vi "Add Unknown Type.vi"(0 "JSON Tree out (JSON Object) in":variant, 5 "result":variant, 9 "Name":string, 11 "error in (no error)":errorcluster) -> (4 "JSON Tree out (JSON Object) out":variant, 15 "error out":errorcluster)   [LabVIEW 2017, in "JSON_RPC_client.lvlib"]
uses:
  JSON_RPC_client.lvlib
  <vilib>/LVH/i3 JSON/JSON Generation/Add Object Parameter Files/Add Object Parameter - String.vi
  <vilib>/LVH/i3 JSON/JSON Generation/Add Object Parameter Files/Add Object Parameter - Object.vi
  <vilib>/LVH/i3 JSON/JSON Generation/Add Object Parameter Files/Add Object Parameter - Array.vi
  <vilib>/LVH/i3 JSON/JSON Generation/Add Object Parameter Files/Add Object Parameter - Boolean.vi
  <vilib>/LVH/i3 JSON/JSON Generation/Add Object Parameter Files/Add Object Parameter - Numeric.vi
  <vilib>/LVH/i3 JSON/JSON Generation/Add Object Parameter Files/Add Object Parameter - 1D Array Boolean.vi
  <vilib>/LVH/i3 JSON/JSON Generation/Add Object Parameter Files/Add Object Parameter - 1D Array String.vi
  <vilib>/LVH/i3 JSON/JSON Generation/Add Object Parameter Files/Add Object Parameter - 1D Array Double.vi
  <vilib>/Utility/Data Type/NI_Data Type.lvlib
  <vilib>/LVH/i3 JSON/i3-json.lvlib
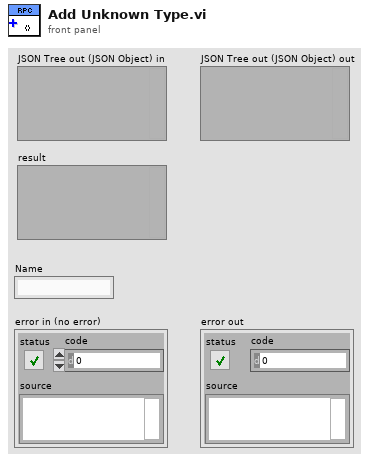
[diagram p1: front panel]
types:
  T1 = typedef "NI_Data Type.lvlib/Data Type.ctl" = enum8{"Invalid Type", "Void", "I8", "I16", "I32", "I64", "U8", "U16", "U32", "U64", "Single Float", "Double Float", "Extended Float", "Single Complex", "Double Complex", "Extended Complex", "Enum U8", "Enum U16", "Enum U32", "Enum U64", "Single Float With Unit", "Double Float With Unit", "Extended Float With Unit", "Single Complex with Unit", "Double Complex with Unit", "Extended Complex with Unit", "Boolean", "String", "Path", "Picture", "Tag", "Array", "Cluster", "Variant", "LV Variant", "Waveform", "Timestamp", "Digital Waveform", "Digital Data", "ExpressData", "Refnum", "External Data", "VI", "Poly VI", "LabVIEW Class Instance", "Fixed Point"}
  T2 = typedef "i3-json.lvlib/JSON Compatible Type.ctl" = enum16{"1D Double Array", "1D String Array", "1D Boolean Array", "Unknown"}
  T3 = typedef "i3-json.lvlib/JSON Type.ctl" = enum8{"JSON Compatible", "JSON Array", "JSON Object", "JSON Null", "Double", "String", "Boolean", "Unknown"}
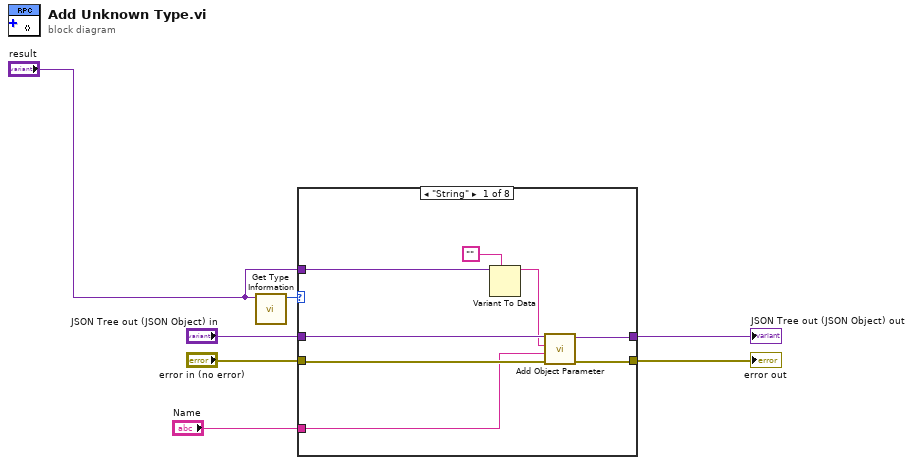
[diagram p0: block diagram]
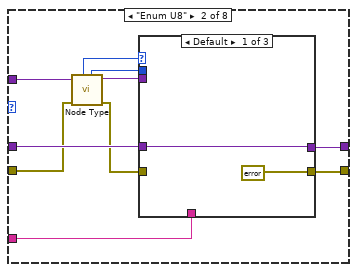
[diagram p2: hidden frame]
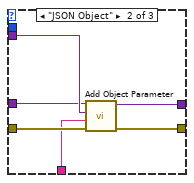
[diagram p3: hidden frame]
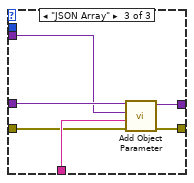
[diagram p4: hidden frame]
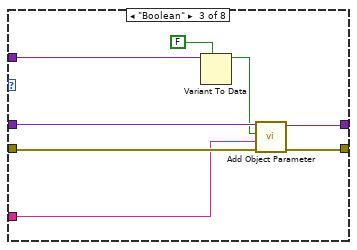
[diagram p5: hidden frame]
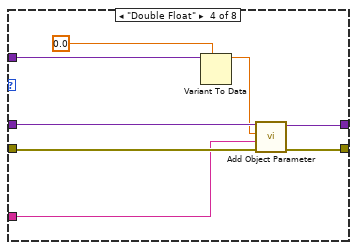
[diagram p6: hidden frame]
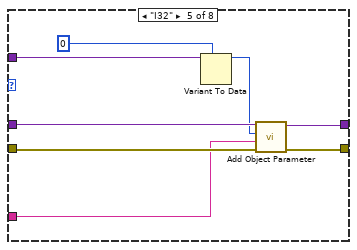
[diagram p7: hidden frame]
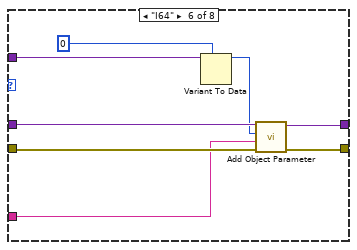
[diagram p8: hidden frame]
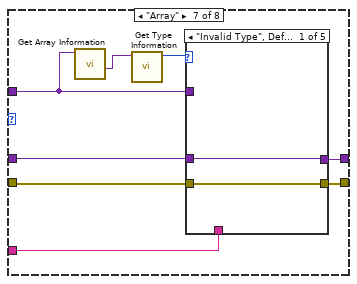
[diagram p9: hidden frame]
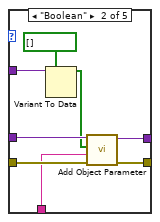
[diagram p10: hidden frame]
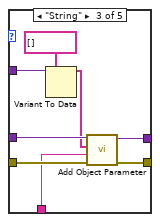
[diagram p11: hidden frame]
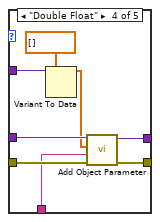
[diagram p12: hidden frame]
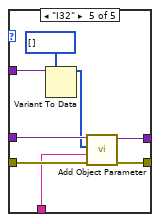
[diagram p13: hidden frame]
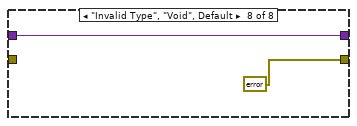
[diagram p14: hidden frame]
diagram:
  n1 = call <vilib>:"Get Type Information.vi"("Variant"="result") -> ("Type"=w6:T1)  [unwired: 6 in, 4 out]
  n2 = case shown="\"String\"" w6 {
    tunnel: "error in (no error)" -> [w12 w20 w44 w52 w60 w68 w76 _]
    tunnel: "JSON Tree out (JSON Object) in" -> [w15 w25 w47 w55 w63 w71 w79 w114]
    tunnel: [w14 w24 w46 w54 w62 w70 w78 w114] -> w3
    tunnel: [w13 w23 w45 w53 w61 w69 w77 errorcluster {"status"=TRUE, "code"=-32603, "source"="JSON-RPC error.  Internal Error.  Result unable to format into JSON.  Ensure the result data type is JSON Object,String, Double, I32, Boolean, or arrays of the same"} ("error constant")] -> w4
    tunnel: "Name" -> [w11 w22 w43 w51 w59 w67 w75 _]
    tunnel: "result" -> [w10 w21 w42 w50 w58 w66 w74 _]
    frame "String" {
      n3 = Variant To Data(type="", Variant=w10) -> (data=w8:string)  [unwired: 1 in, 1 out]
      n4 = call-poly <vilib>:"Add Object Parameter.vi"("error in (no error)"=w12, "Name"=w11, "String"=w8, "JSON Tree in (JSON Object)"=w15) -> ("error out"=w13:errorcluster, "JSON Tree out (JSON Object)"=w14:variant)  [unwired: 6 in]
    }
    frame "Enum U8" {
      n5 = call <vilib>:"Node Type.vi"("error in (no error)"=w20, "JSON Tree In"=w21) -> ("error out"=w19:errorcluster, "JSON Tree Passthrough"=w16:variant, "JSON Compatible Type"=w17:T2, "JSON Type"=w18:T3)  [unwired: 5 in, 1 out]
      n6 = case shown="Default" w18 {
        tunnel: w25 -> [w26 w31 w39]
        tunnel: [w26 w30 w38] -> w24
        tunnel: [errorcluster {"status"=TRUE, "code"=-32603, "source"="JSON-RPC error.  Internal Error.  Result unable to format into JSON.  Ensure the reult data type is JSON Object,String, Double, I32, Boolean, or arrays of the same"} ("error constant") w29 w37] -> w23
        tunnel: w22 -> [_ w28 w36]
        tunnel: w19 -> [_ w33 w35]
        tunnel: w17 -> [_ _ _]
        tunnel: w16 -> [_ w32 w34]
        frame Default {
        }
        frame "JSON Object" {
          n7 = call-poly <vilib>:"Add Object Parameter.vi"("error in (no error)"=w33, "Name"=w28, "JSON Object"=w32, "JSON Tree in (JSON Object)"=w31) -> ("error out"=w29:errorcluster, "JSON Tree out (JSON Object)"=w30:variant)  [unwired: 6 in]
        }
        frame "JSON Array" {
          n8 = call-poly <vilib>:"Add Object Parameter.vi"("error in (no error)"=w35, "Name"=w36, "JSON Array"=w34, "JSON Tree in (JSON Object)"=w39) -> ("error out"=w37:errorcluster, "JSON Tree out (JSON Object)"=w38:variant)  [unwired: 6 in]
        }
      }
    }
    frame "Boolean" {
      n9 = Variant To Data(type=FALSE, Variant=w42) -> (data=w40:bool)  [unwired: 1 in, 1 out]
      n10 = call-poly <vilib>:"Add Object Parameter.vi"("error in (no error)"=w44, "Name"=w43, "Boolean"=w40, "JSON Tree in (JSON Object)"=w47) -> ("error out"=w45:errorcluster, "JSON Tree out (JSON Object)"=w46:variant)  [unwired: 6 in]
    }
    frame "Double Float" {
      n11 = Variant To Data(type=0.0, Variant=w50) -> (data=w48:dbl)  [unwired: 1 in, 1 out]
      n12 = call-poly <vilib>:"Add Object Parameter.vi"("error in (no error)"=w52, "Name"=w51, "Numeric"=w48, "JSON Tree in (JSON Object)"=w55) -> ("error out"=w53:errorcluster, "JSON Tree out (JSON Object)"=w54:variant)  [unwired: 6 in]
    }
    frame "I32" {
      n13 = Variant To Data(type=0, Variant=w58) -> (data=w56:i32)  [unwired: 1 in, 1 out]
      n14 = call-poly <vilib>:"Add Object Parameter.vi"("error in (no error)"=w60, "Name"=w59, "Numeric"=w56, "JSON Tree in (JSON Object)"=w63) -> ("error out"=w61:errorcluster, "JSON Tree out (JSON Object)"=w62:variant)  [unwired: 6 in]
    }
    frame "I64" {
      n15 = Variant To Data(type=0, Variant=w66) -> (data=w64:i32)  [unwired: 1 in, 1 out]
      n16 = call-poly <vilib>:"Add Object Parameter.vi"("error in (no error)"=w68, "Name"=w67, "Numeric"=w64, "JSON Tree in (JSON Object)"=w71) -> ("error out"=w69:errorcluster, "JSON Tree out (JSON Object)"=w70:variant)  [unwired: 6 in]
    }
    frame "Array" {
      n17 = call <vilib>:"Get Array Information.vi"("Variant"=w74) -> ("Array Element Data Type"=w73:variant)  [unwired: 7 in, 3 out]
      n18 = call <vilib>:"Get Type Information.vi"("Variant"=w73) -> ("Type"=w72:T1)  [unwired: 6 in, 4 out]
      n19 = case shown="\"Invalid Type\", Default" w72 {
        tunnel: w79 -> [w81 w89 w97 w105 w113]
        tunnel: [w81 w88 w96 w104 w112] -> w78
        tunnel: [w80 w87 w95 w103 w111] -> w77
        tunnel: w76 -> [w80 w86 w94 w102 w110]
        tunnel: w75 -> [_ w85 w93 w101 w109]
        tunnel: w74 -> [_ w83 w91 w99 w107]
        frame "Invalid Type", Default {
        }
        frame "Boolean" {
          n20 = Variant To Data(type=bool[] [], Variant=w83) -> (data=w84:bool[])  [unwired: 1 in, 1 out]
          n21 = call-poly <vilib>:"Add Object Parameter.vi"("error in (no error)"=w86, "Name"=w85, "1D Boolean"=w84, "JSON Tree in (JSON Object)"=w89) -> ("error out"=w87:errorcluster, "JSON Tree out (JSON Object)"=w88:variant)  [unwired: 6 in]
        }
        frame "String" {
          n22 = Variant To Data(type=string[] [], Variant=w91) -> (data=w92:string[])  [unwired: 1 in, 1 out]
          n23 = call-poly <vilib>:"Add Object Parameter.vi"("error in (no error)"=w94, "Name"=w93, "1D String"=w92, "JSON Tree in (JSON Object)"=w97) -> ("error out"=w95:errorcluster, "JSON Tree out (JSON Object)"=w96:variant)  [unwired: 6 in]
        }
        frame "Double Float" {
          n24 = Variant To Data(type=dbl[] [], Variant=w99) -> (data=w100:dbl[])  [unwired: 1 in, 1 out]
          n25 = call-poly <vilib>:"Add Object Parameter.vi"("error in (no error)"=w102, "Name"=w101, "1D Double"=w100, "JSON Tree in (JSON Object)"=w105) -> ("error out"=w103:errorcluster, "JSON Tree out (JSON Object)"=w104:variant)  [unwired: 6 in]
        }
        frame "I32" {
          n26 = Variant To Data(type=i32[] [], Variant=w107) -> (data=w108:i32[])  [unwired: 1 in, 1 out]
          n27 = call-poly <vilib>:"Add Object Parameter.vi"("error in (no error)"=w110, "Name"=w109, "1D Double"=w108, "JSON Tree in (JSON Object)"=w113) -> ("error out"=w111:errorcluster, "JSON Tree out (JSON Object)"=w112:variant)  [unwired: 6 in]
        }
      }
    }
    frame "Invalid Type", "Void", Default {
    }
  }
  "error out" <- w4
  "JSON Tree out (JSON Object) out" <- w3
